vi "sensor cmd sync dock wait.vi"(11 "device_handle":u32) -> (2 "function return":i32, 3 "device_handle out":u32)   [LabVIEW 2019, in "apdm.lvlib"]
doc: "APDM_EXPORT int apdm_sensor_cmd_sync_dock_wait(apdm_device_handle_t device_handle);"
uses:
  apdm.lvlib
  Lee Lab/CP FES Walking 2018/Code/Working/LabVIEW/apdm.dll
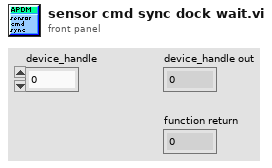
[diagram p1: front panel]
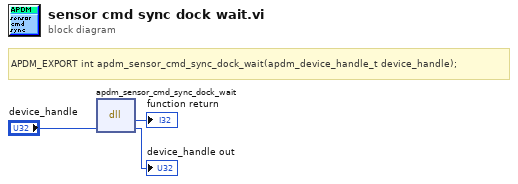
[diagram p0: block diagram]
diagram:
  # "APDM_EXPORT int apdm_sensor_cmd_sync_dock_wait(apdm_device_handle_t device_handle);"
  n1 = dll-call lib="C:/Users/jfalesi/Dropbox/Lee Lab/CP FES Walking 2018/Code/Working/LabVIEW/apdm.*" fn="apdm_sensor_cmd_sync_dock_wait"("device_handle"="device_handle") -> (→"function return":i32, "device_handle"=→"device_handle out":u32)  [unwired: 3 in, 2 out]
